vi "Database_simpletry.vi"() -> ()   [LabVIEW 2012]
uses:
  <vilib>/addons/database/Connection.llb/DB Tools Open Connec (String).vi
  <vilib>/addons/database/NI_Database_API.lvlib
panel:
  out "X-Y Plot":cluster{dbl[], dbl[]}(graph)
  out "data":string[][](table)
  in  "stop":bool
  out "error out":errorcluster
  in  "Table":string
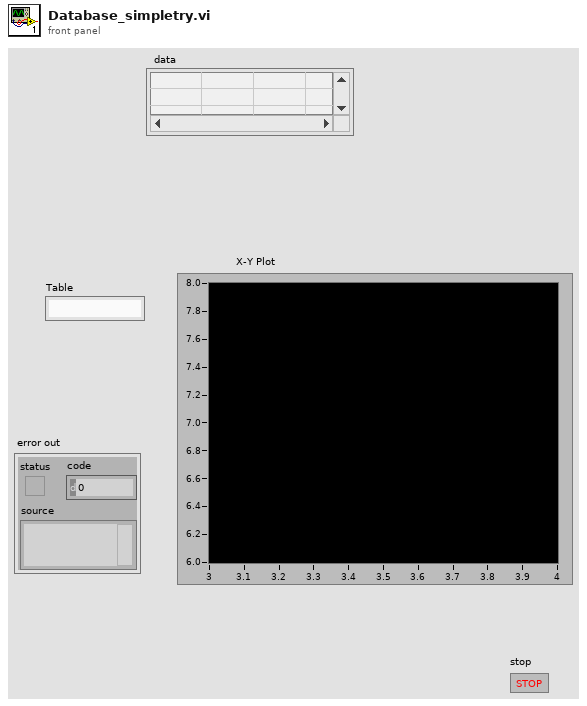
[diagram p1: front panel]
types:
  T1 = typedef "NI_Database_API.lvlib/Conn ObjectReference.ctl" = refnum<k1>
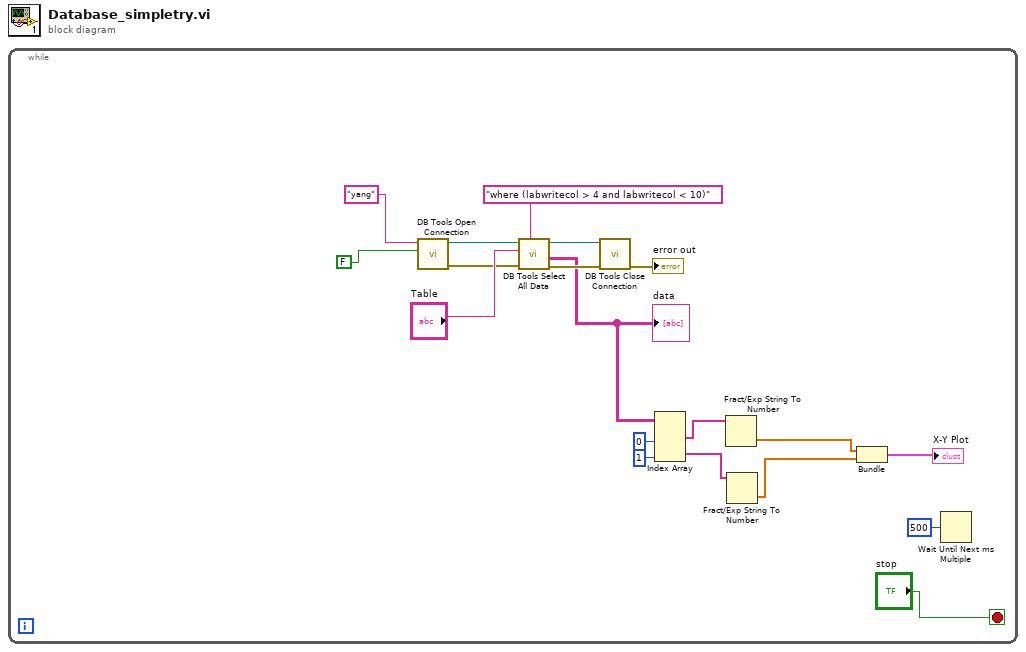
[diagram p0: block diagram]
diagram:
  n1 = while {
    stop <- "stop" stop-if-true
    n2 = call-poly <vilib>:"DB Tools Open Connection.vi"("prompt? (F)"=FALSE, "connection information"="yang" ("condition")) -> ("error out"=w13:errorcluster, "connection reference"=w15:T1)  [unwired: 6 in]
    n3 = call <vilib>:"DB Tools Select All Data.vi"("optional clause"="where (labwritecol > 4 and labwritecol < 10)" ("condition"), "error in (no error)"=w13, "table"="Table", "connection reference"=w15) -> ("error out"=w12:errorcluster, "data"=w9:string[][], "connection reference out"=w11:T1)  [unwired: 1 in, 1 out]
    "data" <- w9
    n4 = call <vilib>:"DB Tools Close Connection.vi"("error in (no error)"=w12, "connection reference"=w11) -> ("error out"=→"error out":errorcluster)  [unwired: 5 in]
    n5 = Index Array(array=w9, index (col) #1=0 ("disabled index (col)"), index (col) #2=1 ("index (col)")) -> (element #1=w6:string[], element #2=w5:string[])  [unwired: 2 in]
    n6 = Fract/Exp String To Number(string=w6) -> (number=w2:dbl[])  [unwired: 4 out]
    n7 = Fract/Exp String To Number(string=w5) -> (number=w4:dbl[])  [unwired: 4 out]
    n8 = Bundle "Bundle"(w2, w4) -> (→"X-Y Plot":cluster{dbl[], dbl[]})  [unwired: 1 in]
    n9 = Wait Until Next ms Multiple(millisecond multiple=u32 500) -> ()  [unwired: 1 out]
  }
